vi "NewFireLauncher.vi"(8 "error in (no error)":errorcluster, 9 "Enum":T1) -> (0 "error out":errorcluster)   [LabVIEW 2013]
uses:
  State Machine Enum.ctl
  <vilib>/Rock Robotics/WPI/Solenoid/WPI_SolenoidValue.ctl
  <vilib>/Rock Robotics/WPI/Solenoid/WPI_SolenoidSetEnum.vi
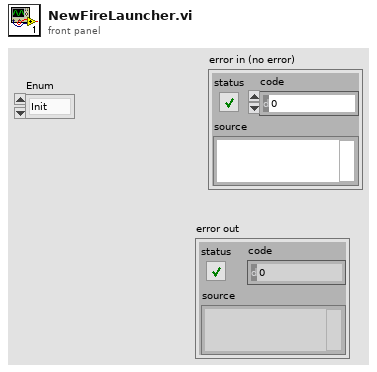
[diagram p1: front panel]
types:
  T1 = typedef "State Machine Enum.ctl" = enum16{"Init", "Actuate", "Retract"}
  T2 = typedef "WPI_SolenoidValue.ctl" = enum16{"Off", "On", "Forward", "Reverse"}
  T3 = typedef "WPI_SolenoidDevRef.ctl" = cluster{"DevStatus":errorcluster, "Solenoid Module":T4, "Forward Solenoid Channel":T5, "Reverse Solenoid Channel":T5}
  T4 = typedef "FPGA_TypedefSolenoidModule.ctl" = enum16{"Solenoid Module 1", "Solenoid Module 2"}
  T5 = typedef "WPI_SolenoidChannel.ctl" = enum8{"Solenoid 1", "Solenoid 2", "Solenoid 3", "Solenoid 4", "Solenoid 5", "Solenoid 6", "Solenoid 7", "Solenoid 8", "Invalid"}
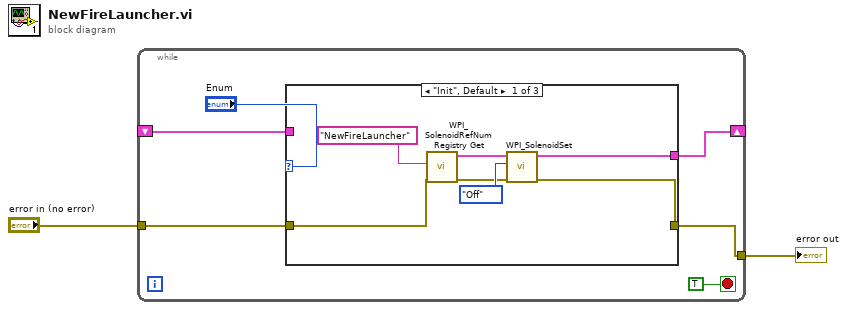
[diagram p0: block diagram]
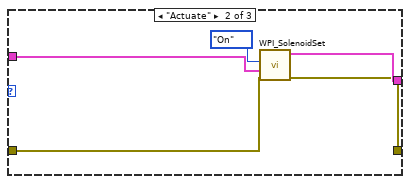
[diagram p2: hidden frame]
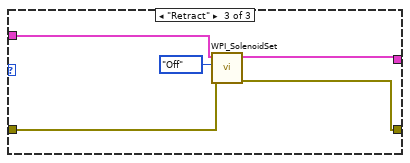
[diagram p3: hidden frame]
diagram:
  n1 = while {
    shift-right: [w6] -> _
    shift-left: _ -> [w5]
    tunnel: "error in (no error)" -> [w4]
    tunnel: [w3] -> w1
    stop <- TRUE stop-if-true
    n2 = case shown="\"Init\", Default" "Enum" {
      tunnel: [w13 w19 w24] -> w6
      tunnel: w5 -> [_ w20 w25]
      tunnel: w4 -> [w11 w17 w22]
      tunnel: [w9 w16 w21] -> w3
      frame "Init", Default {
        n3 = call <vilib>:"WPI_SolenoidRefNum Registry Get.vi"("error in (no error)"=w11, "refnum name"="NewFireLauncher") -> ("error out"=w10:errorcluster, "SolenoidDevRef"=w14:T3)  [unwired: 8 in]
        n4 = call-poly <vilib>:"WPI_SolenoidSet.vi"("error in (no error)"=w10, "Value"=WPI_SolenoidValue."Off", "SolenoidDevRef"=w14) -> ("error out"=w9:errorcluster, "SolenoidDevRef"=w13:T3)  [unwired: 7 in]
      }
      frame "Actuate" {
        n5 = call-poly <vilib>:"WPI_SolenoidSet.vi"("error in (no error)"=w17, "Value"=WPI_SolenoidValue."On", "SolenoidDevRef"=w20) -> ("error out"=w16:errorcluster, "SolenoidDevRef"=w19:T3)  [unwired: 7 in]
      }
      frame "Retract" {
        n6 = call-poly <vilib>:"WPI_SolenoidSet.vi"("error in (no error)"=w22, "Value"=WPI_SolenoidValue."Off", "SolenoidDevRef"=w25) -> ("error out"=w21:errorcluster, "SolenoidDevRef"=w24:T3)  [unwired: 7 in]
      }
    }
  }
  "error out" <- w1
